vi "Interferometer Final.vi"() -> ()   [LabVIEW 2015]
uses:
  <vilib>/Analysis/baseanly.llb/Mean (DBL).vi
  <vilib>/Analysis/NI_AALBase.lvlib
  <vilib>/gmath/NI_Gmath.lvlib
panel:
  in  "WinDaq":refnum<k7>(container)
  out "System State":T1(ring)
  in  "Exit Analysis":bool
  out "Interference":dbl[](array[numeric])
  out "Time":dbl[](array[numeric])
  out "Normalized Delta-T":cluster{dbl[], dbl[]}(graph)
  out "Fourier Transform":T2(graph)
  out "Delta-T":dbl
  out "Detector Values":cluster{dbl[], dbl[]}[](graph)
  out "Interference":cluster{dbl[], dbl[]}(graph)
  out "Channel Count":i32
  in  "Target Channel":i32=2
  in  "Base Channel":i32=1
  in  "Incidence Angle":dbl=25.0
  in  "Wavelength (nm)":dbl=632.2
  out "+/- Error (micron)":dbl
  out "Thickness (micron)":dbl
  out "refnum out":refnum<file>
  in  "Finish Collection":bool
  in  "Time Average Toggle":bool
  out "Cycle Length (s)":dbl
  in  "Measurements per Average":i32=5
  in  "Sample Rate (ms)":i32=100
  in  "Record Buton":bool
  in  "Read Button":bool
  in  "Exit":bool
  out "SaveLocation":path=path "SaveLocation"
  in  "Filename":path
  in  "Directory":path
  # "Interferometer Control"
  # "Startup\n1)  Start DATAQ Hardware Manager\n2) Wait for diodes to be detected\n3) Select Instrument\n4) Press Start WinDaq\n5) Run the Interferometer Final VI"
  # "Time Averaging"
  # "Notes\n1) Keep the cycle lengths to ~ 1s since ice growths take long. If cycle length is shorter than ~1s, time between data aquisition points will slowly grow. This is due to the fourier transform, as it will take longer calculate the FT for a larger dataset. Precise tracking of time between data collection is denoted by Delta T.\n2) Error is determined by the FWHM of the Fourier transform of the interference pattern. The fourier transform is automatically calculated with a left bound denoted by the cursor on the interference graph. Use smaller incidence angles for more precise error calculation. More wavelengths leads to more precise error calculations.\n3) Thickness is automatically saved to the data file. You can find it at the end of the file. Thickness is calculated and saved once the Finish Collection button is pressed. During the Data Analysis stage, you cannot change the value of thickness on the saved file, but you can re-calculate the thickness using the same procedure as when you are measuring."
  # "System Parameters"
  # "Instructions\n1) Enter file folder in directory, and a new filename if \nyou are recording.\n2) Enter system parameters and time averaging parameters to your preferences (reccomended 1s cycle length).\n2) Click  Record to create a new file.\n3) Adjust Left Bound cursor to denote when water deposition \nbegins. Thickness is shown on the left.\n4) Adjust FWHM cursor to the half amplitude of the\nfourier transform to determine error.\n5) Click Finish Collection when you are finished. Data and thickness are automatically saved to the file.\n6) Click Stop Analysis when you are finished analyzing the data.\n7) To view previous data, click Read File and select the desired file.\n8) Adjust Left Bound and FWHM  to recalculate the ice thickness (note: this value does not save) \n9) Click Stop Analysis when you are finished analyzing the data.\n10) Click Exit to stop program."
  # "Channels"
  # "Miscelaneous (System only)"
  # "Keyboard Shortcuts\nRead File -> F1               Record -> F3\nStop Analysis -> F2        Finish Collection -> F4\nTime Average Toggle -> F5        Exit -> Esc\nTime Average -> Page Up/Down"
  # "Pay no attention to the man \nbehind the curtian!"
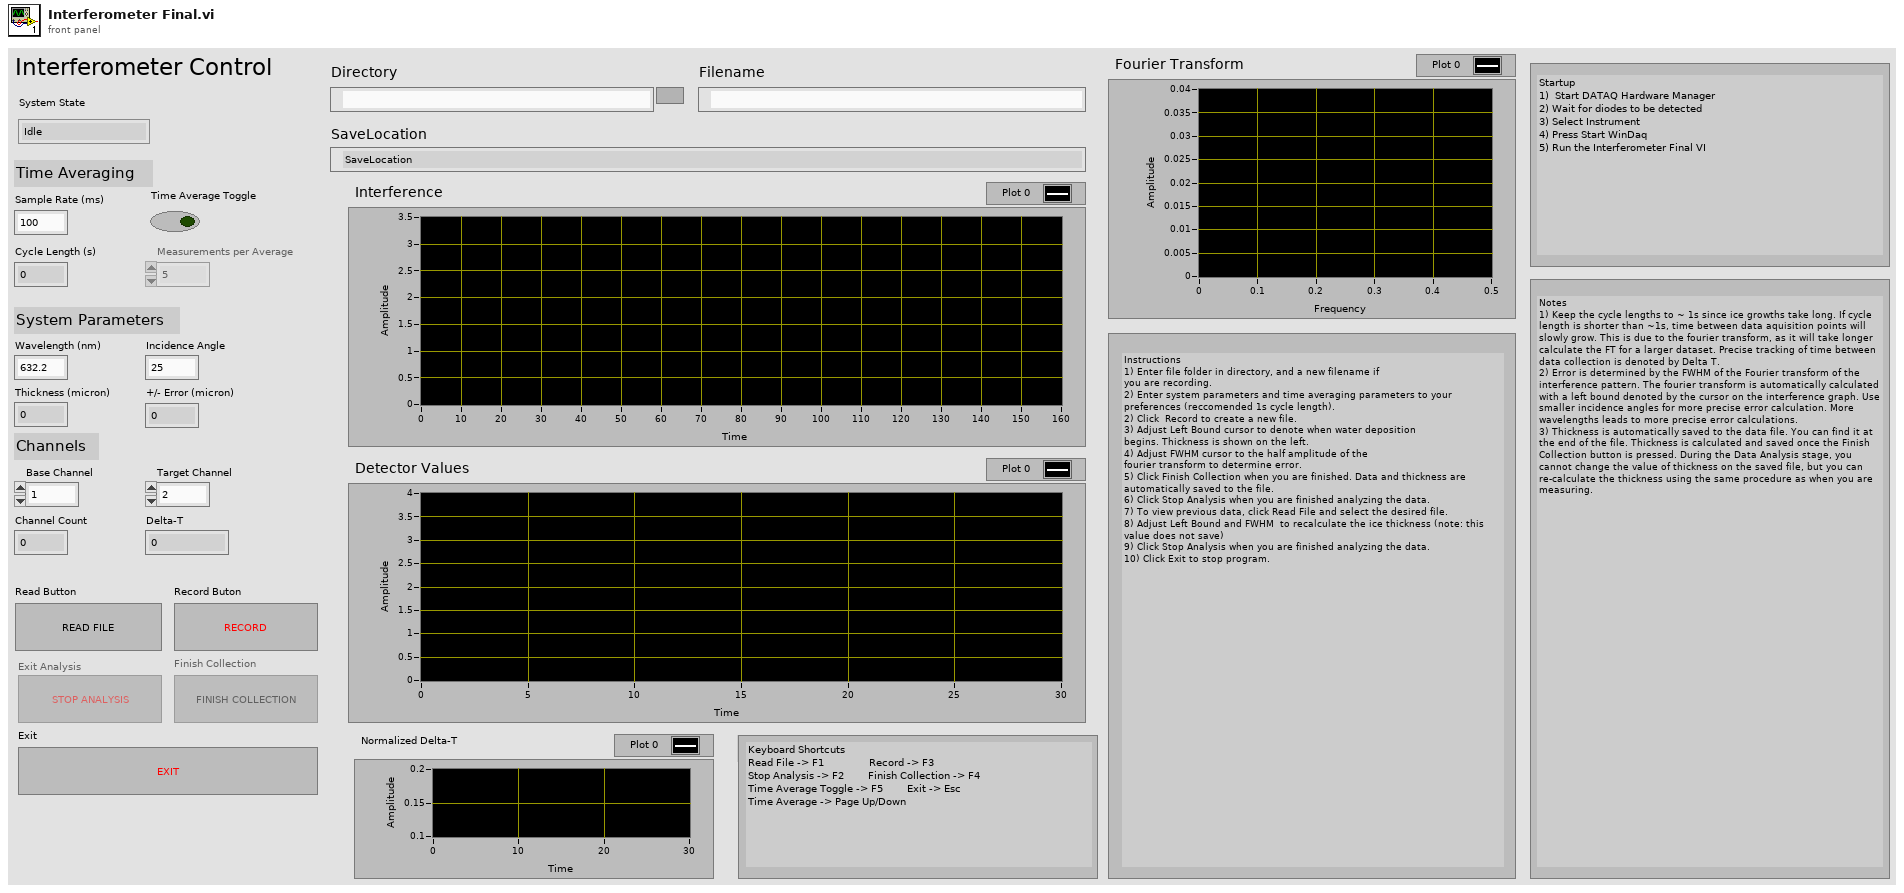
[diagram p1: front panel]
types:
  T1 = enum16{"Idle", "Initialize", "Reset", "Collecting...", "Saving...", "Data Processing", "File Read"}
  T2 = cluster{"Power Spectrum FFT {X} Frequency":dbl[], "Power Spectrum FFT {X}":dbl[]}
  T3 = enum8{"Enabled", "Disabled", "Disabled and Grayed Out"}
  T4 = enum16{"open", "replace", "create", "open or create", "replace or create", "replace or create with confirmation"}
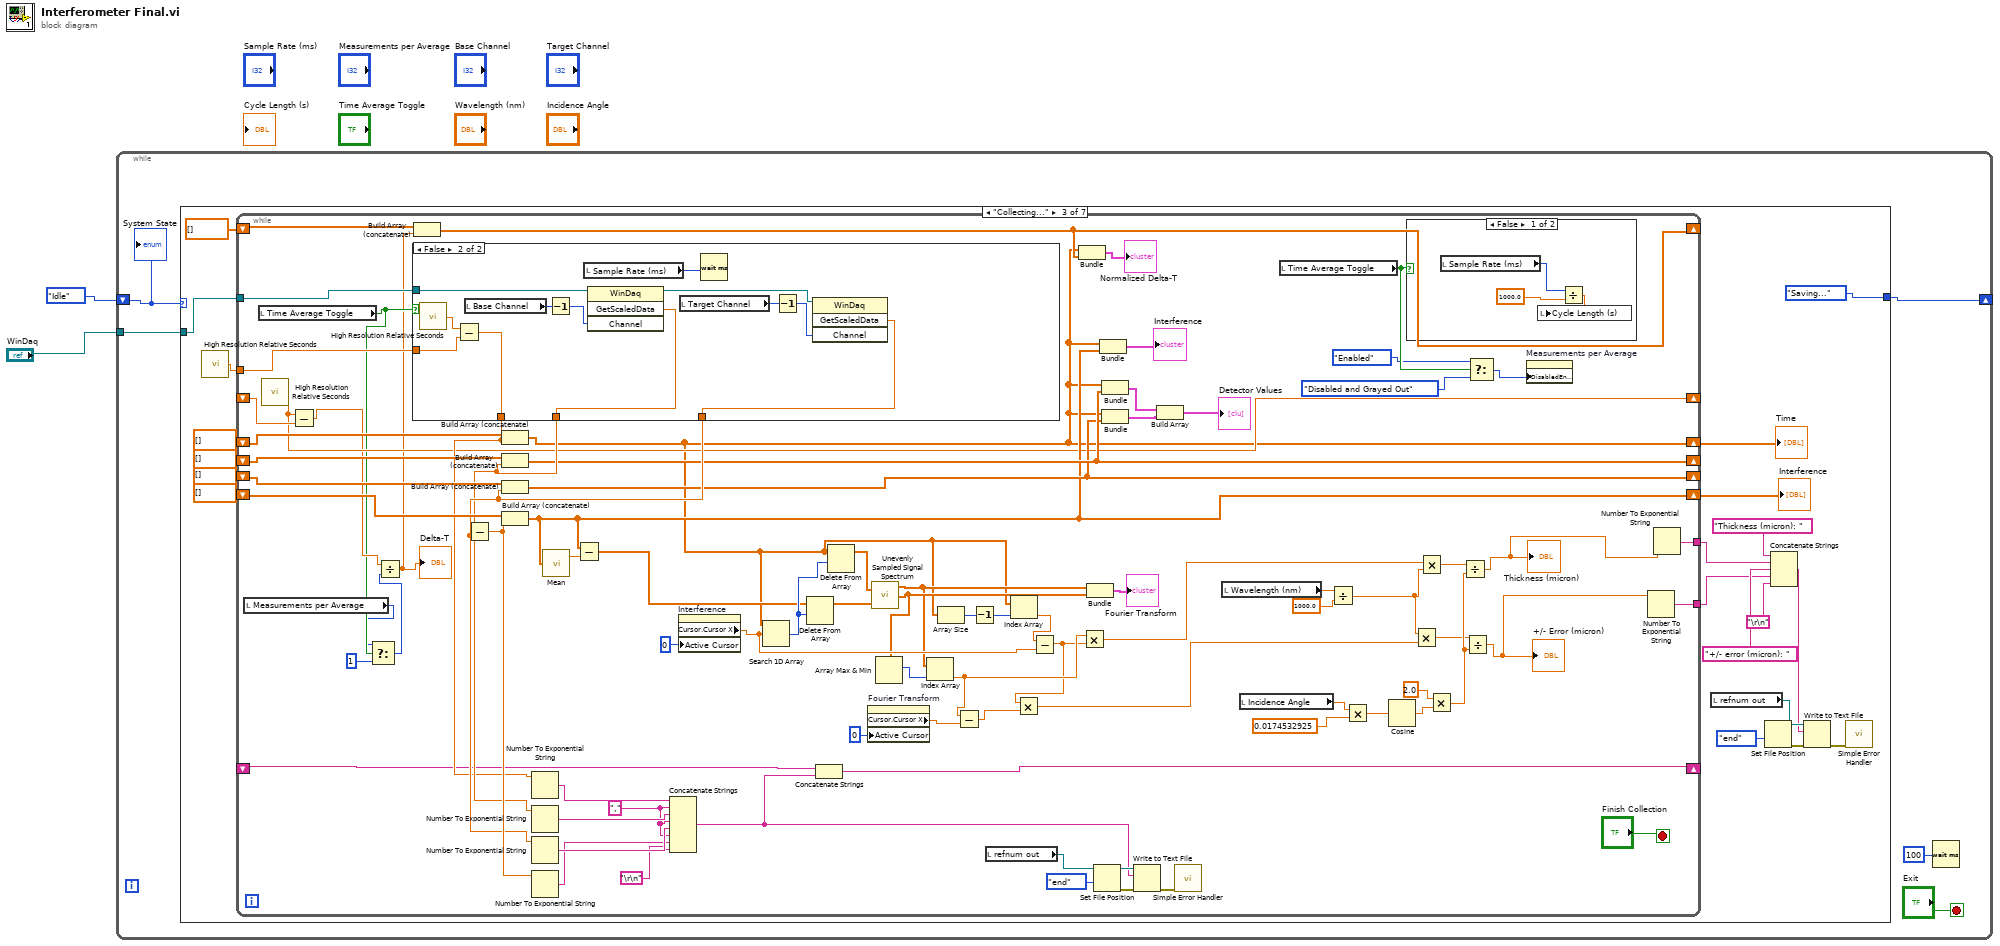
[diagram p0: block diagram]
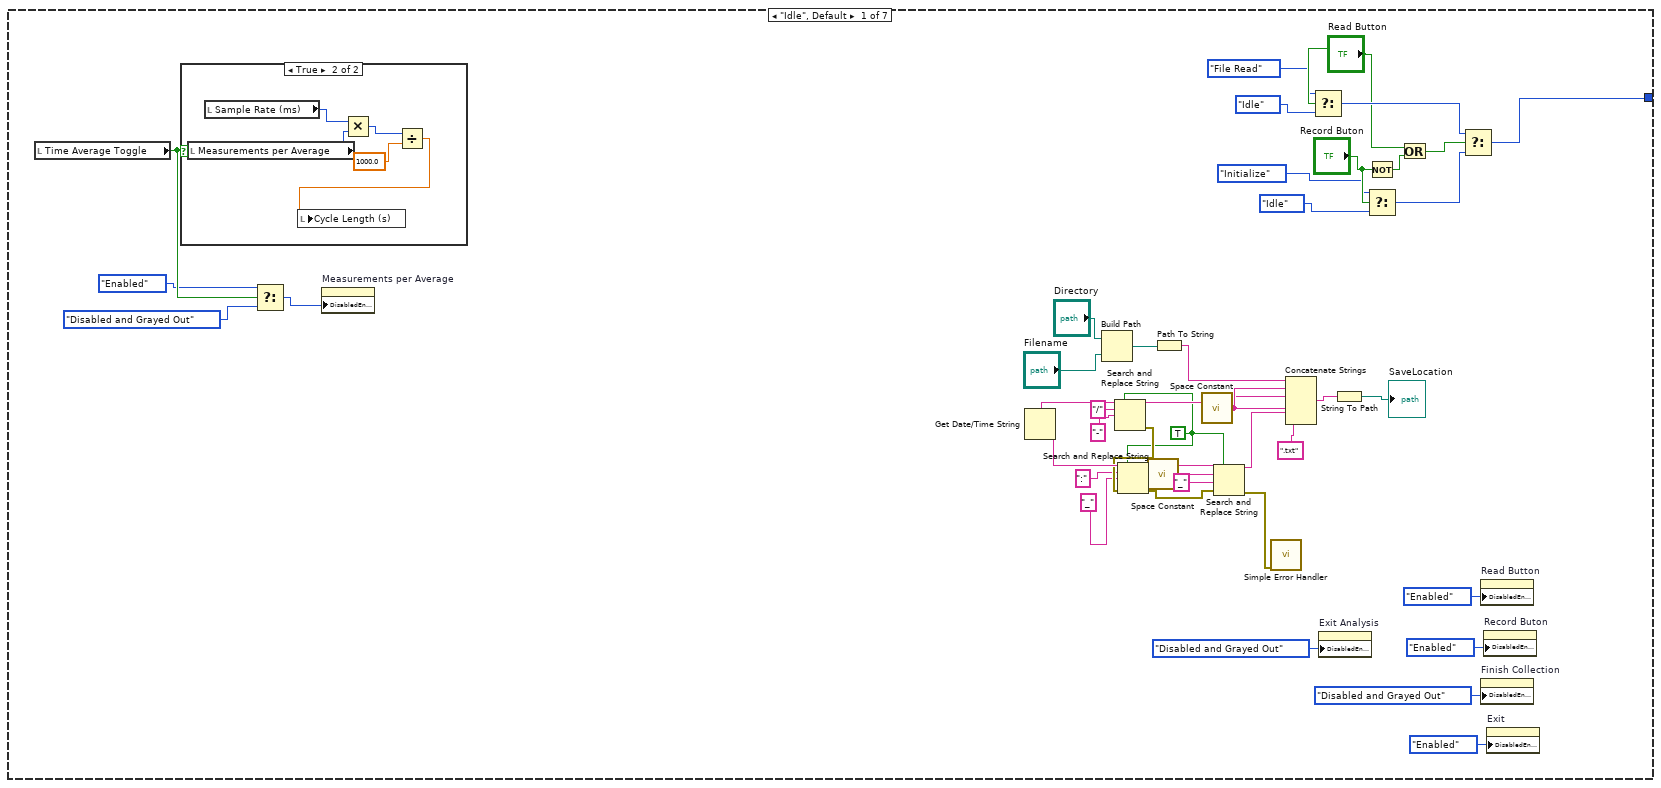
[diagram p2: hidden frame]
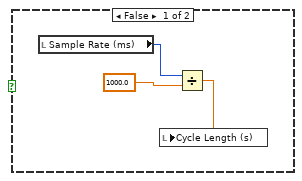
[diagram p3: hidden frame]
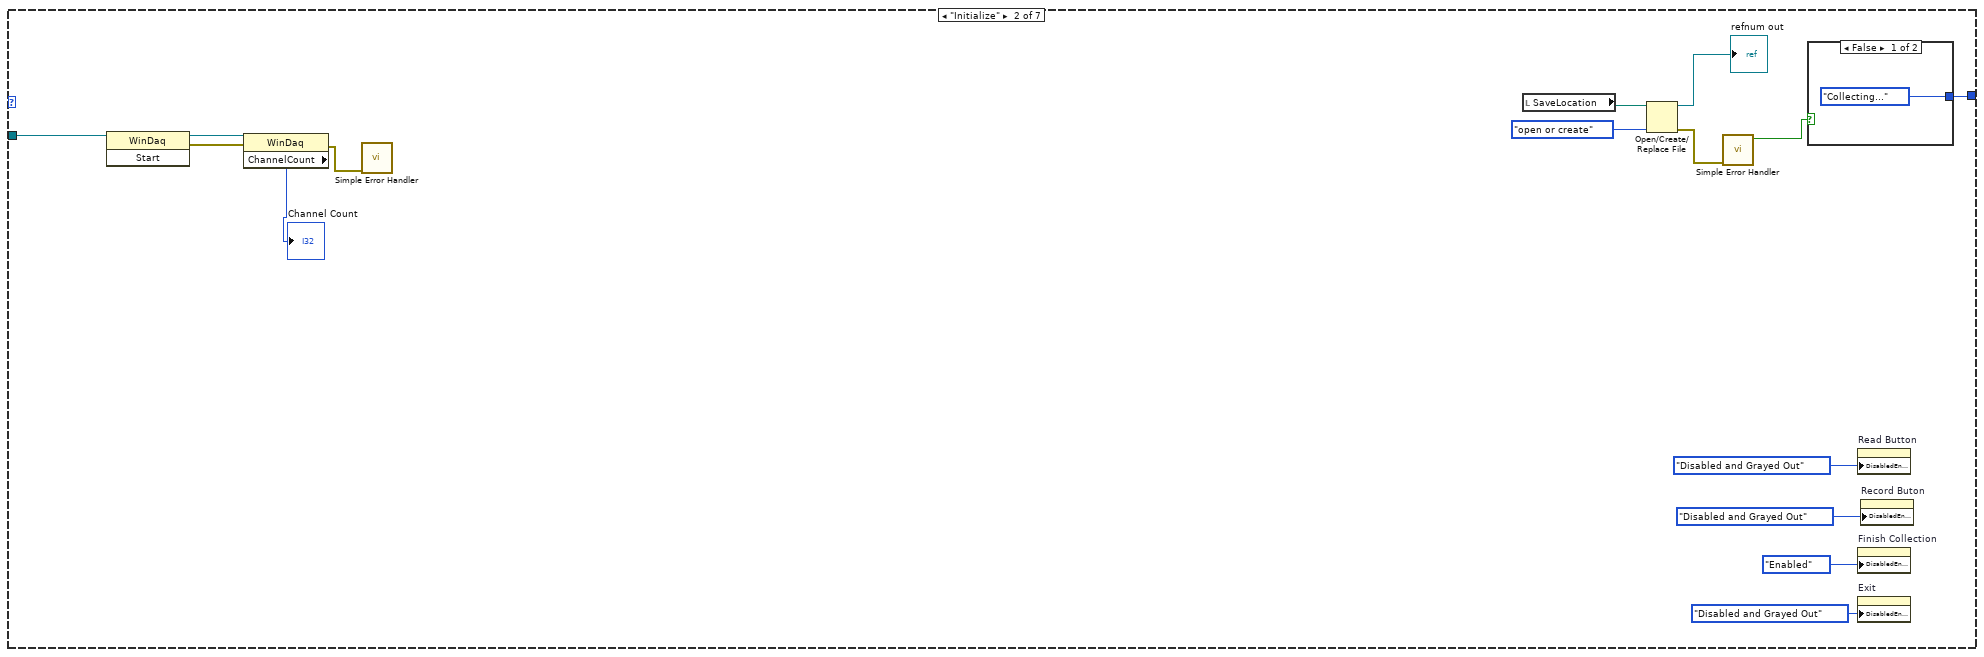
[diagram p4: hidden frame]
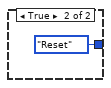
[diagram p5: hidden frame]
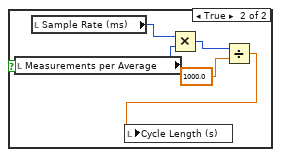
[diagram p6: hidden frame]
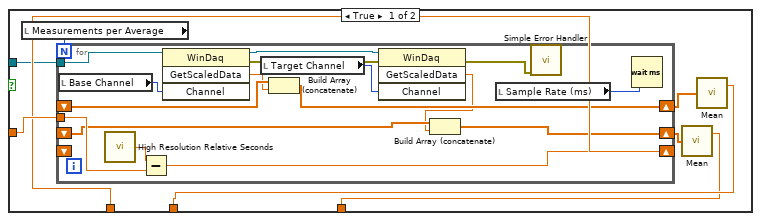
[diagram p7: hidden frame]
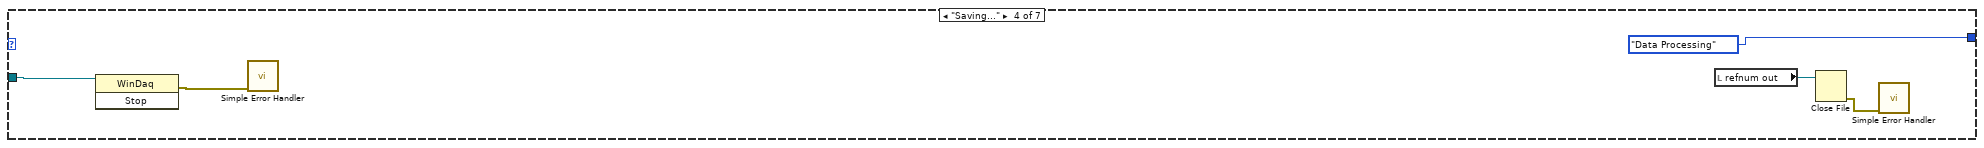
[diagram p8: hidden frame]
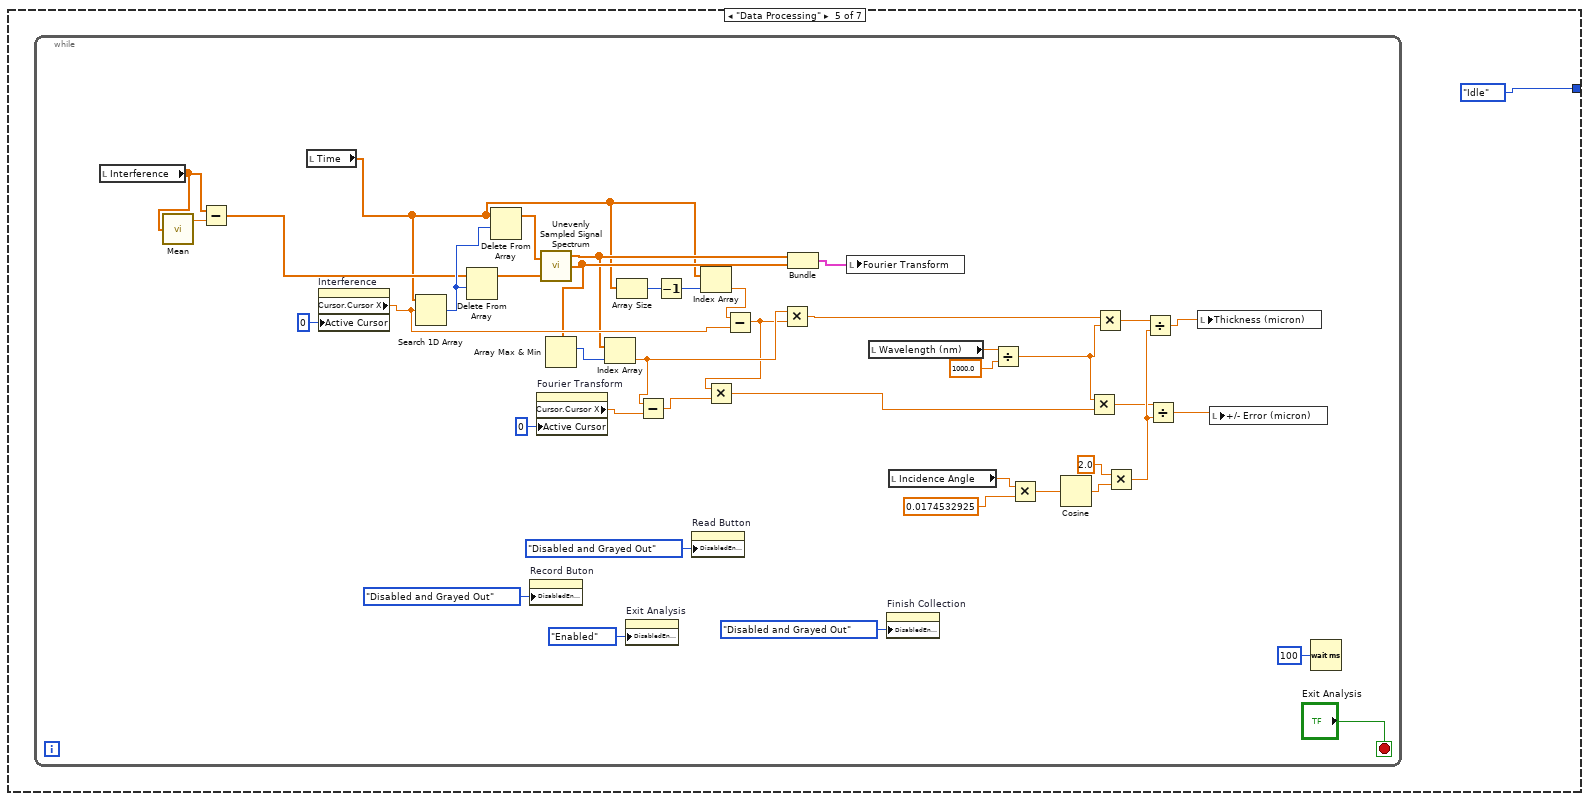
[diagram p9: hidden frame]
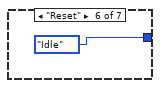
[diagram p10: hidden frame]
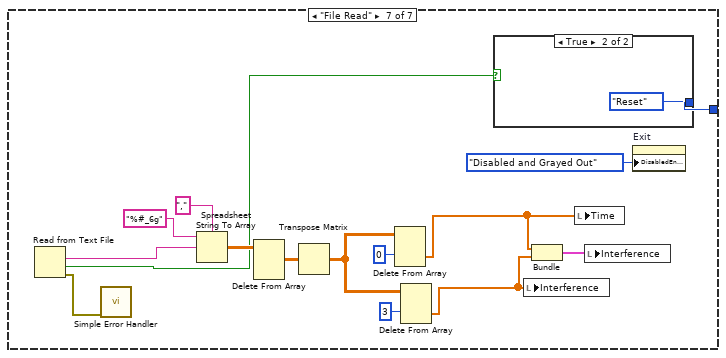
[diagram p11: hidden frame]
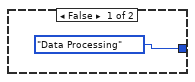
[diagram p12: hidden frame]
diagram:
  n1 = while {
    shift-right: [w4] -> _
    shift-left: T1."Idle" ("Enum") -> [w5]
    tunnel: "WinDaq" -> [w3]
    stop <- "Exit" stop-if-true
    n2 = case shown="\"Collecting...\"" w5 {
      tunnel: [w44 w65 T1."Saving..." ("Enum") T1."Data Processing" ("Enum") T1."Idle" ("Enum") T1."Idle" ("Enum") w288] -> w4
      tunnel: w3 -> [_ w63 w76 w226 _ _ _]
      frame "Idle", Default {
        w28 = TRUE
        n3 = local read "Time Average Toggle"() -> (w18:bool)
        n4 = case shown="True" w18 {
          frame False {
            n5 = local read "Sample Rate (ms)"() -> (w53:i32)
            n6 = Divide(x=w53, y=1000.0) -> (x/y=w51:dbl)
            n7 = local write "Cycle Length (s)"(w51) -> ()
          }
          frame True {
            n8 = local read "Measurements per Average"() -> (w57:i32)
            n9 = local read "Sample Rate (ms)"() -> (w58:i32)
            n10 = Multiply(x=w58, y=w57) -> (x*y=w56:i32)
            n11 = Divide(x=w56, y=1000.0) -> (x/y=w54:dbl)
            n12 = local write "Cycle Length (s)"(w54) -> ()
          }
        }
        n13 = Select(t=T3."Enabled" ("Disabled"), s=w18, f=T3."Disabled and Grayed Out" ("Disabled")) -> (s? t:f=w19:T3)
        n14 = property on="Measurements per Average" class="DigNum (strict)"("DisabledEnum"=w19) -> ()  [unwired: 2 in, 2 out]
        n15 = Get Date/Time String() -> (date string=w30:string, time string=w32:string)  [unwired: 3 in]
        n16 = Build Path(base path="Directory", name or relative path="Filename") -> (appended path=w35:path)
        n17 = Search and Replace String(replace all?=w28, input string=w30, search string="/", replace string="-" ("replace string (\"\")")) -> (result string=w39:string, error out=w31:errorcluster)  [unwired: 4 in, 2 out]
        n18 = Search and Replace String(replace all?=w28, input string=w32, search string=":", replace string="_" ("replace string (\"\")"), error in=w31) -> (result string=w33:string, error out=w34:errorcluster)  [unwired: 3 in, 2 out]
        n19 = call <vilib>:"Space Constant.vi"() -> ("String"=w38:string)
        n20 = Path To String(path=w35) -> (string=w37:string)
        n21 = call <vilib>:"Space Constant.vi"() -> ("String"=w40:string)
        n22 = Search and Replace String(replace all?=w28, input string=w33, search string=w38, replace string="_" ("replace string (\"\")"), error in=w34) -> (result string=w41:string, error out=w36:errorcluster)  [unwired: 3 in, 2 out]
        n23 = call <vilib>:"Simple Error Handler.vi"("error in (no error)"=w36) -> ()  [unwired: 4 in, 5 out]
        n24 = Concatenate Strings(w37, w40, w39, w40, w41, ".txt" ("string")) -> (w42:string)
        n25 = Select(t=T1."File Read" ("Enum"), s="Read Button", f=T1."Idle" ("Enum")) -> (s? t:f=w49:T1)
        n26 = property on="Exit Analysis" class="Bool"("DisabledEnum"=T3."Disabled and Grayed Out" ("Disabled")) -> ()  [unwired: 2 in, 2 out]
        n27 = String To Path(string=w42) -> (path=→"SaveLocation":path)
        n28 = Not(x="Record Buton") -> (.not. x?=w47:bool)
        n29 = Select(t=T1."Initialize" ("Enum"), s="Record Buton", f=T1."Idle" ("Enum")) -> (s? t:f=w50:T1)
        n30 = Or(x="Read Button", y=w47) -> (x .or. y?=w45:bool)
        n31 = Select(t=w49, s=w45, f=w50) -> (s? t:f=w44:T1)
        n32 = property on="Read Button" class="Bool"("DisabledEnum"=T3."Enabled" ("Disabled")) -> ()  [unwired: 2 in, 2 out]
        n33 = property on="Finish Collection" class="Bool"("DisabledEnum"=T3."Disabled and Grayed Out" ("Disabled")) -> ()  [unwired: 2 in, 2 out]
        n34 = property on="Record Buton" class="Bool"("DisabledEnum"=T3."Enabled" ("Disabled")) -> ()  [unwired: 2 in, 2 out]
        n35 = property on="Exit" class="Bool"("DisabledEnum"=T3."Enabled" ("Disabled")) -> ()  [unwired: 2 in, 2 out]
      }
      frame "Initialize" {
        n36 = invoke class="WinDaq" method="Start"(reference=w63) -> (reference out=w62:refnum<k7>, error out=w61:errorcluster)  [unwired: 2 in, 1 out]
        n37 = property class="WinDaq"(reference=w62, error in=w61) -> (error out=w60:errorcluster, "ChannelCount"=→"Channel Count":i16)  [unwired: 1 out]
        n38 = call <vilib>:"Simple Error Handler.vi"("error in (no error)"=w60) -> ()  [unwired: 4 in, 5 out]
        n39 = local read "SaveLocation"() -> (w69:path)
        n40 = Open/Create/Replace File(file path (use dialog)=w69, operation (0:open)=T4."open or create") -> (refnum out=→"refnum out":refnum<file>, error out=w68:errorcluster)  [unwired: 4 in, 1 out]
        n41 = call <vilib>:"Simple Error Handler.vi"("error in (no error)"=w68) -> ("error?"=w64:bool)  [unwired: 4 in, 4 out]
        n42 = case shown="False" w64 {
          tunnel: [T1."Collecting..." ("Enum") T1."Reset" ("Enum")] -> w65
          frame False {
          }
          frame True {
          }
        }
        n43 = property on="Read Button" class="Bool"("DisabledEnum"=T3."Disabled and Grayed Out" ("Disabled")) -> ()  [unwired: 2 in, 2 out]
        n44 = property on="Finish Collection" class="Bool"("DisabledEnum"=T3."Enabled" ("Disabled")) -> ()  [unwired: 2 in, 2 out]
        n45 = property on="Exit" class="Bool"("DisabledEnum"=T3."Disabled and Grayed Out" ("Disabled")) -> ()  [unwired: 2 in, 2 out]
        n46 = property on="Record Buton" class="Bool"("DisabledEnum"=T3."Disabled and Grayed Out" ("Disabled")) -> ()  [unwired: 2 in, 2 out]
      }
      frame "Collecting..." {
        n47 = call <vilib>:"High Resolution Relative Seconds.vi"() -> ("relative seconds"=w96:dbl)
        n48 = while {
          shift-right: [w104] -> w78
          shift-left: dbl[] [] -> [w176]
          shift-right: [w156] -> _
          shift-left: dbl[] [] -> [w175]
          shift-right: [w155] -> _
          shift-left: dbl[] [] -> [w174]
          tunnel: w96 -> [w149]
          shift-right: [w154] -> w79
          shift-left: dbl[] [] -> [w172]
          shift-right: [w160] -> _
          shift-left: _ -> [w159]
          shift-right: [w147] -> _
          shift-left: _ -> [w148]
          shift-right: [w109] -> _
          shift-left: dbl[] [] -> [w111]
          tunnel: [w106] -> w87
          tunnel: [w105] -> w89
          tunnel: w76 -> [w103]
          stop <- "Finish Collection" stop-if-true
          w164 = ","
          n49 = local read "Measurements per Average"() -> (w99:i32)
          n50 = local read "Time Average Toggle"() -> (w100:bool)
          n51 = call <vilib>:"High Resolution Relative Seconds.vi"() -> ("relative seconds"=w147:dbl)
          n52 = Subtract(x=w147, y=w148) -> (x-y=w101:dbl)
          n53 = Select(t=w99, s=w100, f=1) -> (s? t:f=w102:i32)
          n54 = Divide(x=w101, y=w102) -> (x/y=w97:dbl)
          "Delta-T" <- w97
          n55 = case shown="False" w100 {
            tunnel: w149 -> [w195 w223]
            tunnel: [w191 w213] -> w170
            tunnel: [w190 w214] -> w168
            tunnel: [w192 w220] -> w169
            tunnel: w103 -> [w189 w218]
            frame True {
              n56 = local read "Measurements per Average"() -> (w196:i32)
              n57 = for {
                N: w196 -> [_]
                shift-right: [w209] -> w194
                shift-left: _ -> [w207]
                shift-right: [w205] -> w190
                shift-left: _ -> [_]
                shift-right: [w210] -> w193
                shift-left: _ -> [w208]
                tunnel: w195 -> [w211]
                tunnel: w189 -> [w204]
                n58 = local read "Base Channel"() -> (w202:i32)
                n59 = call <vilib>:"High Resolution Relative Seconds.vi"() -> ("relative seconds"=w212:dbl)
                n60 = Subtract(x=w212, y=w211) -> (x-y=w205:dbl)
                n61 = invoke class="WinDaq" method="GetScaledData"(reference=w204, "Channel"=w202) -> (reference out=w199:refnum<k7>, error out=w198:errorcluster, "GetScaledData"=w203:dbl)  [unwired: 2 in, 1 out]
                n62 = local read "Target Channel"() -> (w200:i32)
                n63 = Build Array (concatenate)(w208, w203) -> (w210:dbl[])
                n64 = invoke class="WinDaq" method="GetScaledData"(reference=w199, error in=w198, "Channel"=w200) -> (error out=w197:errorcluster, "GetScaledData"=w201:dbl)  [unwired: 1 in, 2 out]
                n65 = Build Array (concatenate)(w207, w201) -> (w209:dbl[])
                n66 = local read "Sample Rate (ms)"() -> (w206:i32)
                n67 = call <vilib>:"Simple Error Handler.vi"("error in (no error)"=w197) -> ()  [unwired: 4 in, 5 out]
                n68 = Wait (ms)(milliseconds to wait=w206) -> ()  [unwired: 1 out]
              }
              n69 = call-poly <vilib>:"Mean.vi"("X"=w194) -> ("mean"=w191:dbl)  [unwired: 1 out]
              n70 = call-poly <vilib>:"Mean.vi"("X"=w193) -> ("mean"=w192:dbl)  [unwired: 1 out]
            }
            frame False {
              n71 = call <vilib>:"High Resolution Relative Seconds.vi"() -> ("relative seconds"=w224:dbl)
              n72 = Subtract(x=w224, y=w223) -> (x-y=w214:dbl)
              n73 = local read "Base Channel"() -> (w221:i32)
              n74 = Decrement(x=w221) -> (x-1=w215:i32)
              n75 = local read "Sample Rate (ms)"() -> (w222:i32)
              n76 = invoke class="WinDaq" method="GetScaledData"(reference=w218, "Channel"=w215) -> (reference out=w219:refnum<k7>, "GetScaledData"=w220:dbl)  [unwired: 2 in, 2 out]
              n77 = local read "Target Channel"() -> (w217:i32)
              n78 = Wait (ms)(milliseconds to wait=w222) -> ()  [unwired: 1 out]
              n79 = Decrement(x=w217) -> (x-1=w216:i32)
              n80 = invoke class="WinDaq" method="GetScaledData"(reference=w219, "Channel"=w216) -> ("GetScaledData"=w213:dbl)  [unwired: 2 in, 3 out]
            }
          }
          n81 = Build Array (concatenate)(w111, w97) -> (w109:dbl[])
          n82 = Subtract(x=w169, y=w170) -> (x-y=w171:dbl)
          n83 = Build Array (concatenate)(w176, w168) -> (w104:dbl[])
          n84 = Build Array (concatenate)(w175, w169) -> (w156:dbl[])
          n85 = Build Array (concatenate)(w174, w170) -> (w155:dbl[])
          n86 = Build Array (concatenate)(w172, w171) -> (w154:dbl[])
          n87 = Number To Exponential String(number=w168) -> (E-format string=w167:string)  [unwired: 3 in]
          n88 = Number To Exponential String(number=w169) -> (E-format string=w166:string)  [unwired: 3 in]
          n89 = Number To Exponential String(number=w170) -> (E-format string=w165:string)  [unwired: 3 in]
          n90 = Number To Exponential String(number=w171) -> (E-format string=w163:string)  [unwired: 3 in]
          n91 = call-poly <vilib>:"Mean.vi"("X"=w154) -> ("mean"=w157:dbl)  [unwired: 1 out]
          n92 = Subtract(x=w154, y=w157) -> (x-y=w120:dbl[])
          n93 = Concatenate Strings(w167, w164, w166, w164, w165, w164, w163, "\r\n") -> (w161:string)
          n94 = property on="Interference" class="XYGraph (strict)"("Active Cursor"=u32 0) -> ("Cursor.Cursor X"=w139:dbl)  [unwired: 2 in, 2 out]
          n95 = Search 1D Array(1D array=w104, element=w139) -> (index of element=w142:i32)  [unwired: 1 in]
          n96 = Delete From Array(array=w120, length=w142) -> (array with subset deleted=w141:dbl[])  [unwired: 1 in, 1 out]
          n97 = Concatenate Strings(w159, w161) -> (w160:string)
          n98 = Delete From Array(array=w104, length=w142) -> (array with subset deleted=w125:dbl[])  [unwired: 1 in, 1 out]
          n99 = property on="Fourier Transform" class="XYGraph (strict)"("Active Cursor"=u32 0) -> ("Cursor.Cursor X"=w115:dbl)  [unwired: 2 in, 2 out]
          n100 = call <vilib>:"Unevenly Sampled Signal Spectrum.vi"("XTime"=w125, "X"=w141) -> ("Power Spectrum FFT {X} Frequency"=w118:dbl[], "Power Spectrum FFT {X}"=w119:dbl[])  [unwired: 1 out]
          n101 = Array Max & Min(array=w119) -> (max index (indices)=w131:i32)  [unwired: 3 out]
          n102 = Index Array(array=w118, index=w131) -> (element=w116:dbl)
          n103 = Array Size(array=w104) -> (size(s)=w134:i32)
          n104 = Subtract(x=w116, y=w115) -> (x-y=w113:dbl)
          n105 = Decrement(x=w134) -> (x-1=w133:i32)
          n106 = local read "refnum out"() -> (w158:refnum<file>)
          n107 = Index Array(array=w104, index=w133) -> (element=w132:dbl)
          n108 = Subtract(x=w132, y=w139) -> (x-y=w114:dbl)
          n109 = Multiply(x=w114, y=w113) -> (x*y=w112:dbl)
          n110 = Bundle(w104, w109) -> (→"Normalized Delta-T":cluster{dbl[], dbl[]})  [unwired: 1 in]
          n111 = Multiply(x=w116, y=w114) -> (x*y=w129:dbl)
          n112 = Bundle("Power Spectrum FFT {X} Frequency"=w118, "Power Spectrum FFT {X}"=w119) -> (→"Fourier Transform":T2)  [unwired: 1 in]
          n113 = Set File Position(refnum=w158, from (0:start)=enum16{"start", "end", "current"}."end") -> (refnum out=w179:refnum<file>, error out=w178:errorcluster)  [unwired: 2 in]
          n114 = Bundle(w104, w154) -> (→"Interference":cluster{dbl[], dbl[]})  [unwired: 1 in]
          n115 = Bundle(w104, w156) -> (w153:cluster{dbl[], dbl[]})  [unwired: 1 in]
          n116 = Bundle(w104, w155) -> (w152:cluster{dbl[], dbl[]})  [unwired: 1 in]
          n117 = Write to Text File(file (use dialog)=w179, text=w161, error in=w178) -> (error out=w177:errorcluster)  [unwired: 1 in, 2 out]
          n118 = Build Array(w153, w152) -> (→"Detector Values":cluster{dbl[], dbl[]}[])
          n119 = call <vilib>:"Simple Error Handler.vi"("error in (no error)"=w177) -> ()  [unwired: 4 in, 5 out]
          n120 = local read "Wavelength (nm)"() -> (w130:dbl)
          n121 = local read "Incidence Angle"() -> (w137:dbl)
          n122 = local read "Time Average Toggle"() -> (w145:bool)
          n123 = Divide(x=w130, y=1000.0) -> (x/y=w127:dbl)
          n124 = Multiply(x=w137, y=0.0174532925) -> (x*y=w138:dbl)
          n125 = Cosine(x=w138) -> (cos(x)=w136:dbl)
          n126 = case shown="False" w145 {
            frame False {
              n127 = local read "Sample Rate (ms)"() -> (w183:i32)
              n128 = Divide(x=w183, y=1000.0) -> (x/y=w181:dbl)
              n129 = local write "Cycle Length (s)"(w181) -> ()
            }
            frame True {
              n130 = local read "Measurements per Average"() -> (w187:i32)
              n131 = local read "Sample Rate (ms)"() -> (w188:i32)
              n132 = Multiply(x=w188, y=w187) -> (x*y=w186:i32)
              n133 = Divide(x=w186, y=1000.0) -> (x/y=w184:dbl)
              n134 = local write "Cycle Length (s)"(w184) -> ()
            }
          }
          n135 = Multiply(x=w127, y=w112) -> (x*y=w126:dbl)
          n136 = Multiply(x=w129, y=w127) -> (x*y=w128:dbl)
          n137 = Multiply(x=2.0, y=w136) -> (x*y=w135:dbl)
          n138 = Divide(x=w128, y=w135) -> (x/y=w108:dbl)
          "Thickness (micron)" <- w108
          n139 = Divide(x=w126, y=w135) -> (x/y=w107:dbl)
          "+/- Error (micron)" <- w107
          n140 = Select(t=T3."Enabled" ("Disabled"), s=w145, f=T3."Disabled and Grayed Out" ("Disabled")) -> (s? t:f=w146:T3)
          n141 = property on="Measurements per Average" class="DigNum (strict)"("DisabledEnum"=w146) -> ()  [unwired: 2 in, 2 out]
          n142 = Number To Exponential String(number=w107) -> (E-format string=w106:string)  [unwired: 3 in]
          n143 = Number To Exponential String(number=w108) -> (E-format string=w105:string)  [unwired: 3 in]
        }
        "Time" <- w78
        "Interference" <- w79
        n144 = local read "refnum out"() -> (w85:refnum<file>)
        n145 = Set File Position(refnum=w85, from (0:start)=enum16{"start", "end", "current"}."end") -> (refnum out=w82:refnum<file>, error out=w83:errorcluster)  [unwired: 2 in]
        n146 = Concatenate Strings("Thickness (micron): ", w89, "+/- error (micron): ", w87, "\r\n") -> (w80:string)
        n147 = Write to Text File(file (use dialog)=w82, text=w80, error in=w83) -> (error out=w84:errorcluster)  [unwired: 1 in, 2 out]
        n148 = call <vilib>:"Simple Error Handler.vi"("error in (no error)"=w84) -> ()  [unwired: 4 in, 5 out]
      }
      frame "Saving..." {
        n149 = invoke class="WinDaq" method="Stop"(reference=w226) -> (error out=w225:errorcluster)  [unwired: 2 in, 2 out]
        n150 = call <vilib>:"Simple Error Handler.vi"("error in (no error)"=w225) -> ()  [unwired: 4 in, 5 out]
        n151 = local read "refnum out"() -> (w229:refnum<file>)
        n152 = Close File(refnum=w229) -> (error out=w228:errorcluster)  [unwired: 1 in, 1 out]
        n153 = call <vilib>:"Simple Error Handler.vi"("error in (no error)"=w228) -> ()  [unwired: 4 in, 5 out]
      }
      frame "Data Processing" {
        n154 = while {
          stop <- "Exit Analysis" stop-if-true
          n155 = local read "Interference"() -> (w254:dbl[])
          n156 = call-poly <vilib>:"Mean.vi"("X"=w254) -> ("mean"=w272:dbl)  [unwired: 1 out]
          n157 = Subtract(x=w254, y=w272) -> (x-y=w263:dbl[])
          n158 = local read "Time"() -> (w235:dbl[])
          n159 = property on="Interference" class="XYGraph (strict)"("Active Cursor"=u32 0) -> ("Cursor.Cursor X"=w269:dbl)  [unwired: 2 in, 2 out]
          n160 = Search 1D Array(1D array=w235, element=w269) -> (index of element=w271:i32)  [unwired: 1 in]
          n161 = Delete From Array(array=w263, length=w271) -> (array with subset deleted=w270:dbl[])  [unwired: 1 in, 1 out]
          n162 = Delete From Array(array=w235, length=w271) -> (array with subset deleted=w264:dbl[])  [unwired: 1 in, 1 out]
          n163 = property on="Record Buton" class="Bool"("DisabledEnum"=T3."Disabled and Grayed Out" ("Disabled")) -> ()  [unwired: 2 in, 2 out]
          n164 = property on="Fourier Transform" class="XYGraph (strict)"("Active Cursor"=u32 0) -> ("Cursor.Cursor X"=w259:dbl)  [unwired: 2 in, 2 out]
          n165 = call <vilib>:"Unevenly Sampled Signal Spectrum.vi"("XTime"=w264, "X"=w270) -> ("Power Spectrum FFT {X} Frequency"=w261:dbl[], "Power Spectrum FFT {X}"=w262:dbl[])  [unwired: 1 out]
          n166 = Array Max & Min(array=w262) -> (max index (indices)=w265:i32)  [unwired: 3 out]
          n167 = Index Array(array=w261, index=w265) -> (element=w260:dbl)
          n168 = Array Size(array=w235) -> (size(s)=w268:i32)
          n169 = property on="Exit Analysis" class="Bool"("DisabledEnum"=T3."Enabled" ("Disabled")) -> ()  [unwired: 2 in, 2 out]
          n170 = Subtract(x=w260, y=w259) -> (x-y=w257:dbl)
          n171 = Decrement(x=w268) -> (x-1=w267:i32)
          n172 = property on="Read Button" class="Bool"("DisabledEnum"=T3."Disabled and Grayed Out" ("Disabled")) -> ()  [unwired: 2 in, 2 out]
          n173 = Index Array(array=w235, index=w267) -> (element=w266:dbl)
          n174 = Subtract(x=w266, y=w269) -> (x-y=w258:dbl)
          n175 = Multiply(x=w258, y=w257) -> (x*y=w241:dbl)
          n176 = Multiply(x=w260, y=w258) -> (x*y=w242:dbl)
          n177 = Bundle("Power Spectrum FFT {X} Frequency"=w261, "Power Spectrum FFT {X}"=w262) -> (w236:T2)  [unwired: 1 in]
          n178 = local write "Fourier Transform"(w236) -> ()
          n179 = local read "Wavelength (nm)"() -> (w249:dbl)
          n180 = property on="Finish Collection" class="Bool"("DisabledEnum"=T3."Disabled and Grayed Out" ("Disabled")) -> ()  [unwired: 2 in, 2 out]
          n181 = local read "Incidence Angle"() -> (w252:dbl)
          n182 = Divide(x=w249, y=1000.0) -> (x/y=w247:dbl)
          n183 = Multiply(x=w252, y=0.0174532925) -> (x*y=w253:dbl)
          n184 = Cosine(x=w253) -> (cos(x)=w251:dbl)
          n185 = Multiply(x=w247, y=w241) -> (x*y=w246:dbl)
          n186 = Multiply(x=w242, y=w247) -> (x*y=w248:dbl)
          n187 = Multiply(x=2.0, y=w251) -> (x*y=w250:dbl)
          n188 = Divide(x=w248, y=w250) -> (x/y=w240:dbl)
          n189 = Divide(x=w246, y=w250) -> (x/y=w239:dbl)
          n190 = local write "Thickness (micron)"(w240) -> ()
          n191 = local write "+/- Error (micron)"(w239) -> ()
          n192 = Wait (ms)(milliseconds to wait=u32 100) -> ()  [unwired: 1 out]
        }
      }
      frame "Reset" {
      }
      frame "File Read" {
        n193 = Read from Text File() -> (text=w286:string, cancelled=w275:bool, error out=w274:errorcluster)  [unwired: 4 in, 1 out]
        n194 = call <vilib>:"Simple Error Handler.vi"("error in (no error)"=w274) -> ()  [unwired: 4 in, 5 out]
        n195 = Spreadsheet String To Array(delimiter (Tab)=",", format string="%#_6g", spreadsheet string=w286) -> (array=w282:dbl[][])  [unwired: 1 in]
        n196 = Delete From Array(array=w282) -> (array with subset deleted=w276:dbl[][])  [unwired: 3 in, 1 out]
        n197 = Transpose Matrix(1:w276) -> (0:w277:dbl[][])
        n198 = Delete From Array(array=w277, index (row)=0) -> (deleted portion=w280:dbl[])  [unwired: 2 in, 1 out]
        n199 = Delete From Array(array=w277, index (row)=3) -> (deleted portion=w279:dbl[])  [unwired: 2 in, 1 out]
        n200 = case shown="True" w275 {
          tunnel: [T1."Data Processing" ("Enum") T1."Reset" ("Enum")] -> w288
          frame False {
          }
          frame True {
          }
        }
        n201 = local write "Interference"(w279) -> ()
        n202 = Bundle(w280, w279) -> (w281:cluster{dbl[], dbl[]})  [unwired: 1 in]
        n203 = local write "Time"(w280) -> ()
        n204 = local write "Interference"(w281) -> ()
        n205 = property on="Exit" class="Bool"("DisabledEnum"=T3."Disabled and Grayed Out" ("Disabled")) -> ()  [unwired: 2 in, 2 out]
      }
    }
    n206 = Wait (ms)(milliseconds to wait=u32 100) -> ()  [unwired: 1 out]
    "System State" <- w5
  }
